vi "S30c_dll F69.vi"(4 "error in":errorcluster, 7 "Dev Addr":u8=250) -> (0 "error out":errorcluster, 2 "Serial number":i32)   [LabVIEW 2014, in "K_S30c_dll.lvlib"]
uses:
  K_S30c_dll.lvlib
  s30c.dll
panel:
  # "Function 69: Read Serial number \nusing s30c.dll\nKeller AG für Druckmesstechnik, 29.5.08 b.v."
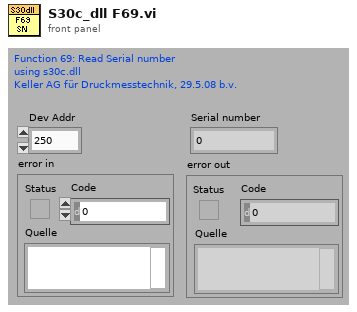
[diagram p1: front panel]
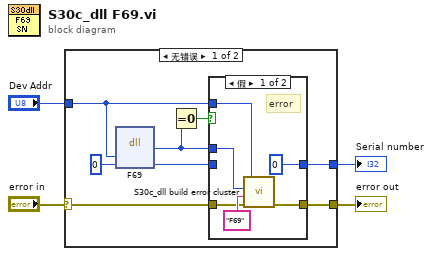
[diagram p0: block diagram]
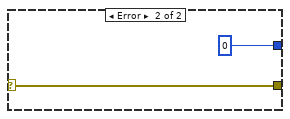
[diagram p3: hidden frame]
diagram:
  n1 = case shown="无错误" "error in" {
    selector: "error in" -> [w10 w22]
    tunnel: "Dev Addr" -> [w7 _]
    tunnel: [w9 w22] -> w3
    tunnel: [w5 0 ("SN")] -> w2
    frame No Error {
      n2 = dll-call lib="PTH2Labs EworkSINOPEC北控自动相渗software2.08.5_dlls30c.dll" fn="F69" label="dll call F69"("DevAddr"=w7, "SN"=0 ("Data")) -> (w8:i16, "SN"=w6:i32)  [unwired: 4 in, 2 out]
      n3 = Equal To 0?(x=w8) -> (x = 0?=w12:bool)
      n4 = case shown="假" w12 {
        tunnel: w10 -> [w17 w19]
        tunnel: [w16 w19] -> w9
        tunnel: w8 -> [w15 _]
        tunnel: w7 -> [w14 _]
        tunnel: w6 -> [_ w20]
        tunnel: [0 ("SN") w20] -> w5
        frame False {
          # "error"
          n5 = call "S30c_dll build error cluster.vi"("error in"=w17, "error Text"="F69", "error code"=w15, "Dev Addr"=w14) -> ("error out"=w16:errorcluster)  [unwired: 3 in]
        }
        frame True {
        }
      }
    }
    frame Error {
    }
  }
  "error out" <- w3
  "Serial number" <- w2
